vi "Submit HTTP Request.vi"(8 "error in":errorcluster, 11 "Data":T1) -> (0 "error out":errorcluster, 3 "Data Out":T1)   [LabVIEW 2014]
uses:
  Controls/Data.ctl
  Controls/FP Control Refs.ctl
  Controls/Property.ctl
  Controls/Address.ctl
  Controls/Filter Criteria.ctl
  Controls/Fields.ctl
  Controls/Operator.ctl
  <vilib>/httpClient/LabVIEWHTTPClient.lvlib
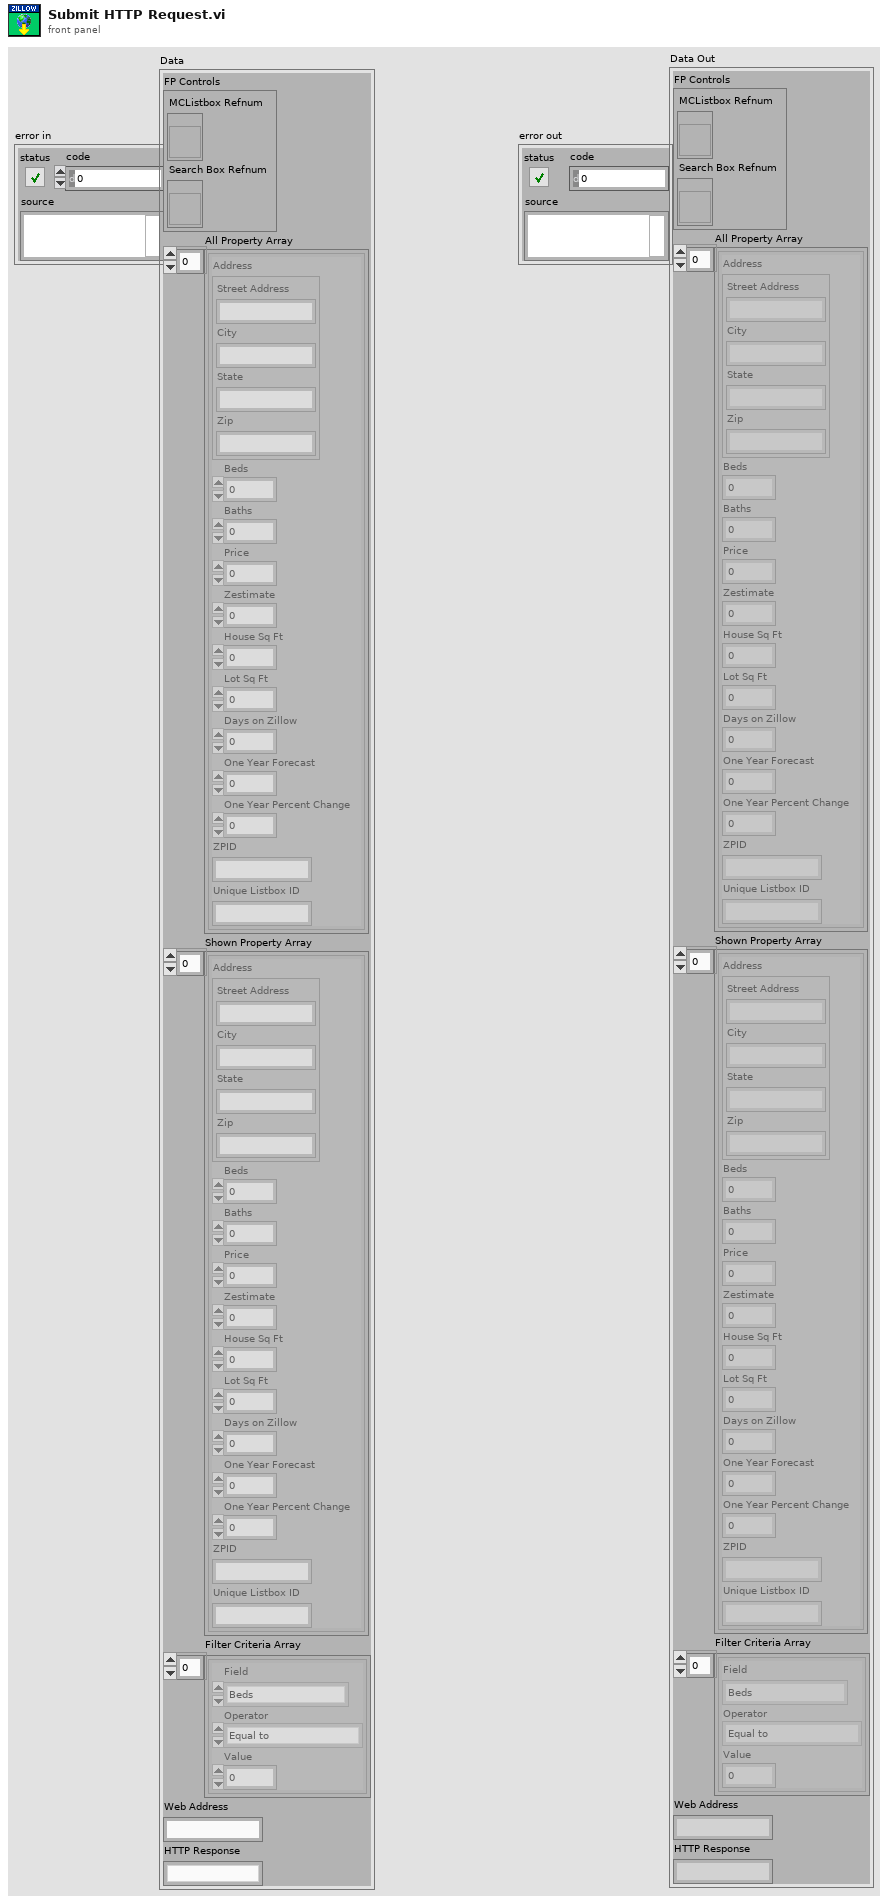
[diagram p1: front panel]
types:
  T1 = typedef "Data.ctl" = cluster{"FP Controls":T2, "All Property Array":T3[], "Shown Property Array":T3[], "Filter Criteria Array":T5[], "Web Address":string, "HTTP Response":string}
  T2 = typedef "FP Control Refs.ctl" = cluster{"MCListbox Refnum":refnum<vi>, "Search Box Refnum":refnum<vi>}
  T3 = typedef "Property.ctl" = cluster{"Address":T4, "Beds":dbl, "Baths":dbl, "Price":dbl, "Zestimate":dbl, "House Sq Ft":dbl, "Lot Sq Ft":dbl, "Days on Zillow":dbl, "One Year Forecast":dbl, "One Year Percent Change":dbl, "ZPID":string, "Unique Listbox ID":string}
  T4 = typedef "Address.ctl" = cluster{"Street Address":string, "City":string, "State":string, "Zip":string}
  T5 = typedef "Filter Criteria.ctl" = cluster{"Field":T6, "Operator":T7, "Value":dbl}
  T6 = typedef "Fields.ctl" = enum16{"Beds", "Baths", "Price", "Zestimate", "House Sq Ft", "Lot Sq Ft", "Days on Zillow", "One Year Forecast", "One Year Percent Change"}
  T7 = typedef "Operator.ctl" = enum16{"Equal to", "Greater than (or equal)", "Less than (or equal)", "Not Equal to"}
  T8 = typedef "LabVIEWHTTPClient.lvlib/ClientHandle.ctl" = refnum<k1>
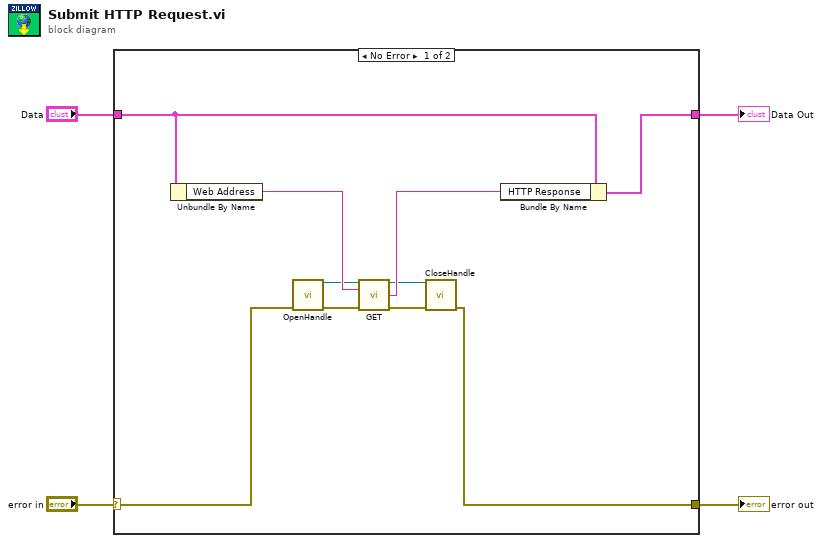
[diagram p0: block diagram]
diagram:
  n1 = case shown="No Error" "error in" {
    selector: "error in" -> [w11 w16]
    tunnel: [w10 w16] -> w3
    tunnel: "Data" -> [w9 w15]
    tunnel: [w14 w15] -> w1
    frame No Error {
      n2 = Unbundle By Name(w9) -> ("Web Address"=w8:string)
      n3 = call <vilib>:"OpenHandle.vi"("error in (no error)"=w11) -> ("client handle out"=w6:T8, "error out"=w13:errorcluster)  [unwired: 13 in]
      n4 = call <vilib>:"GET.vi"("client handle"=w6, "url"=w8, "error in (no error)"=w13) -> ("client handle out"=w5:T8, "body"=w7:string, "error out"=w12:errorcluster)  [unwired: 9 in, 1 out]
      n5 = call <vilib>:"CloseHandle.vi"("client handle"=w5, "error in (no error)"=w12) -> ("error out"=w10:errorcluster)  [unwired: 13 in]
      n6 = Bundle By Name(cluster=w9, "HTTP Response"=w7) -> (w14:T1)
    }
    frame Error {
    }
  }
  "error out" <- w3
  "Data Out" <- w1
